vi "Model Query.vi"(7 "Slave Address":i32=-1 min=-1 max=30 step=1, 8 "error":errorcluster, 11 "VISA":refnum<visa-resource-name>) -> (0 "error out":errorcluster, 1 "Current Rating":dbl format="%.1f", 2 "Voltage Rating":dbl format="%.1f", 3 "VISA out":refnum<visa-resource-name>, 4 "Serial Number":string, 6 "Model":string="GEN<Vrate>-<Irate>-<Option>")   [LabVIEW 2025, in "TDK-Lambda GEN LAN Series.lvlib"]
doc: "Reads the power supply's Identity string and returns:\n\nVoltage Rating: the maximum output voltage (volts)\nCurrent Rating: the maximum output current (amps)\nModel Number: is string, example: \"GEN6-200-LAN\" \nSerial Number: is string, example: \"12C4581AA\""
uses:
  <userlib>/TDK-Lambda GEN LAN Series/TDK-Lambda GEN LAN Series.lvlib
panel:
  # "TDK-Lambda Genesys \n LAN\n  DC Power Supplies"
  # "Read Model Ratings"
  # "GEN<Vrate>-<Irate>-<Option>"
  # "(c) 2019 TDK-Lambda.  ALL RIGHTS RESERVED."
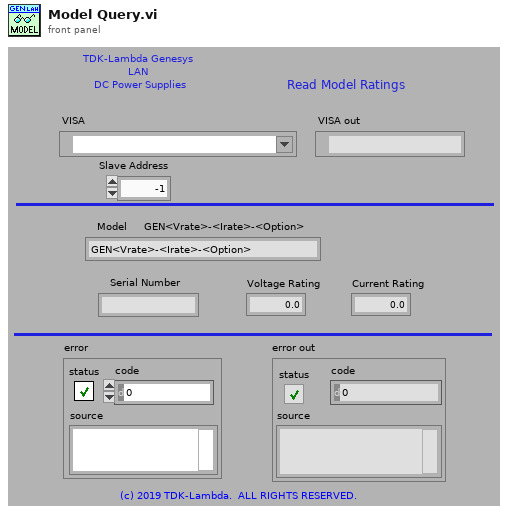
[diagram p1: front panel]
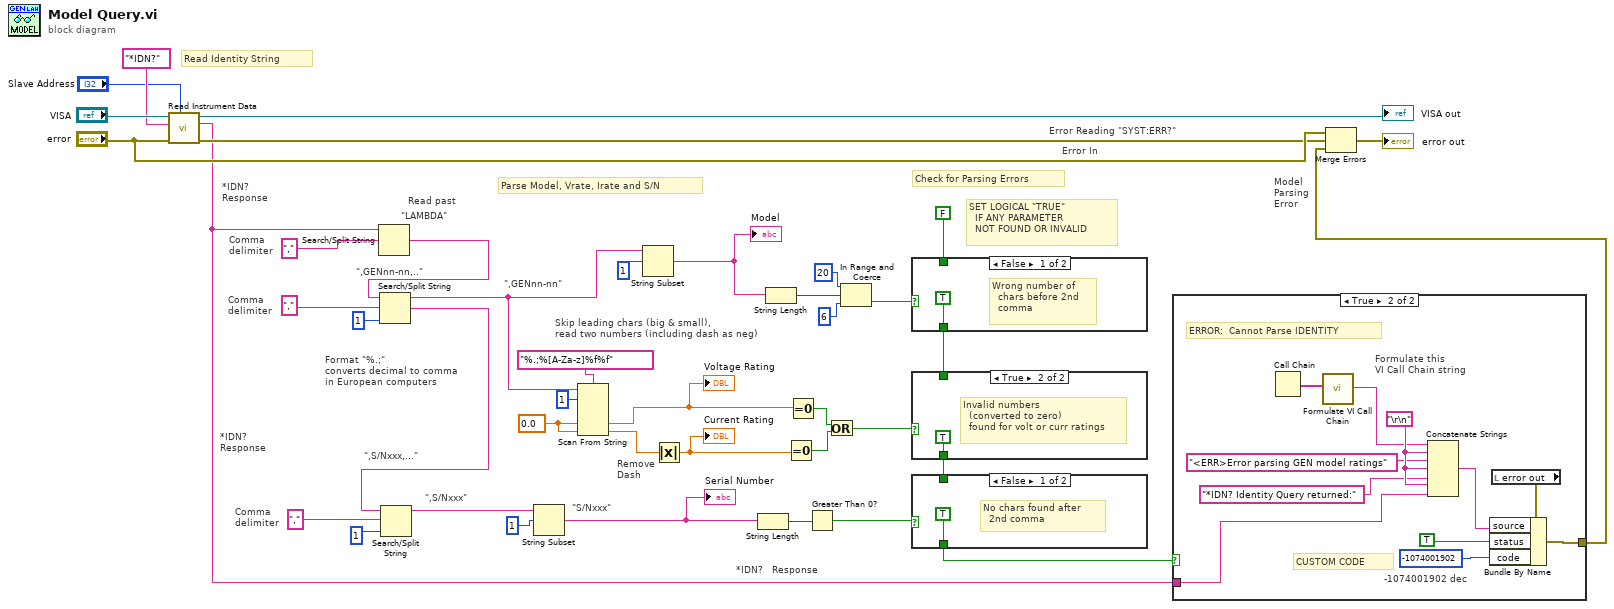
[diagram p0: block diagram]
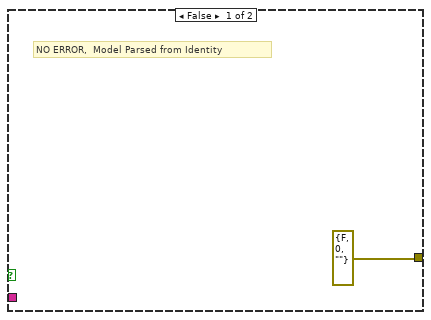
[diagram p5: hidden frame]
diagram:
  w23 = 0.0 ("default value 2")
  # "*IDN?   Response"
  # "*IDN? \nResponse"
  # "Check for Parsing Errors"
  # "Parse Model, Vrate, Irate and S/N"
  # "*IDN? \nResponse"
  # "Read past"
  # "Format \"%.;\"\nconverts decimal to comma\nin European computers"
  # "SET LOGICAL \"TRUE\" \n  IF ANY PARAMETER    \n  NOT FOUND OR INVALID"
  # "Comma\ndelimiter"
  # "Comma\ndelimiter"
  # "Comma\ndelimiter"
  # "\"S/Nxxx\""
  # "\",S/Nxxx\""
  # "Skip leading chars (big & small),\nread two numbers (including dash as neg)"
  # "Remove\nDash"
  # "\",GENnn-nn,..\""
  # "\",GENnn-nn\""
  # "\",S/Nxxx,...\""
  # "\"LAMBDA\""
  # "Model\nParsing\nError"
  # "Error Reading \"SYST:ERR?\""
  # "Error In"
  # "Read Identity String"
  n1 = call <userlib>:"Read Instrument Data.vi"("Slave Address"="Slave Address", "error"="error", "Query"="*IDN?" ("format string"), "VISA"="VISA") -> ("error out"=w37:errorcluster, "Response"=w3:string, "VISA out"=→"VISA out":refnum<visa-resource-name>)  [unwired: 4 in, 1 out]
  n2 = Search/Split String(string=w3, search string/char (-)="," ("format string")) -> (match + rest of string=w35:string)  [unwired: 1 in, 2 out]
  n3 = Search/Split String(string=w35, search string/char (-)="," ("format string"), offset (0)=1) -> (substring before match=w7:string, match + rest of string=w26:string)  [unwired: 1 out]
  n4 = Search/Split String(string=w26, search string/char (-)="," ("format string"), offset (0)=1) -> (substring before match=w25:string)  [unwired: 2 out]
  n5 = String Subset(string=w25, offset (0)=1) -> (substring=w8:string)  [unwired: 1 in]
  "Serial Number" <- w8
  n6 = Scan From String(format string="%.;%[A-Za-z]%f%f", input string=w7, initial scan location=u32 1, default 2=w23, default 3=w23) -> (output 2=w10:dbl, output 3=w32:dbl)  [unwired: 3 in, 3 out]
  "Voltage Rating" <- w10
  n7 = String Subset(string=w7, offset (0)=1) -> (substring=w5:string)  [unwired: 1 in]
  "Model" <- w5
  n8 = Absolute Value(x=w32) -> (abs(x)=w9:dbl)
  "Current Rating" <- w9
  n9 = String Length(string=w8) -> (length=w13:i32)
  n10 = String Length(string=w5) -> (length=w21:i32)
  n11 = Equal To 0?(x=w9) -> (x = 0?=w16:bool)
  n12 = Equal To 0?(x=w10) -> (x = 0?=w17:bool)
  n13 = Greater Than 0?(x=w13) -> (x > 0?=w12:bool)
  n14 = Or(x=w17, y=w16) -> (x .or. y?=w15:bool)
  n15 = In Range and Coerce(upper limit=20, x=w21, lower limit=6) -> (In Range?=w22:bool)  [unwired: 1 out]
  n16 = case shown="False" w22 {
    tunnel: FALSE -> [_ w43]
    tunnel: [TRUE w43] -> w14
    frame False {
      # "Wrong number of\n  chars before 2nd   \n  comma"
    }
    frame True {
      # "Correct number of  \n  chars before 2nd\n  comma"
    }
  }
  n17 = case shown="True" w15 {
    tunnel: w14 -> [w44 _]
    tunnel: [w44 TRUE] -> w11
    frame False {
      # "Valid numbers found  \n  for volt & curr ratings"
    }
    frame True {
      # "Invalid numbers   \n  (converted to zero) \n  found for volt or curr ratings"
    }
  }
  n18 = case shown="False" w12 {
    tunnel: w11 -> [_ w47]
    tunnel: [TRUE w47] -> w4
    frame False {
      # "No chars found after  \n  2nd comma"
    }
    frame True {
      # "At least one char in  \n  serial number field"
    }
  }
  n19 = case shown="True" w4 {
    tunnel: w3 -> [_ w51]
    tunnel: [errorcluster {"status"=FALSE, "code"=0, "source"=""} ("error out") w52] -> w2
    frame False {
      # "NO ERROR,  Model Parsed from Identity"
    }
    frame True {
      w59 = "\r\n"
      # "CUSTOM CODE"
      # "-1074001902 dec"
      # "Formulate this \nVI Call Chain string"
      # "ERROR:  Cannot Parse IDENTITY"
      n20 = Call Chain() -> (call chain=w49:string[])
      n21 = call <userlib>:"Formulate VI Call Chain.vi"("Call Chain"=w49) -> ("String Out"=w50:string)  [unwired: 10 in]
      n22 = Concatenate Strings(w50, w59, "<ERR>Error parsing GEN model ratings" ("Source"), w59, "*IDN? Identity Query returned:" ("Source"), w59, w51) -> (w58:string)
      n23 = local read "error out"() -> (w57:errorcluster)
      n24 = Bundle By Name(cluster=w57, "source"=w58, "status"=TRUE, "code"=-1074001902) -> (w52:errorcluster)
    }
  }
  n25 = Merge Errors("error", w37, w2) -> (→"error out":errorcluster)
